vi "SelectSpectrum.vi"(4 "Following":enum32{"Mag", "Temp", "Last"}(radio), 6 "Param":enum16{"S11", "S21", "S12", "S22"}(ring), 8 "Cursor.Cursor Index":i32, 10 "Data_IN":T1={"Value"=0.0, "GUI Data Cluster"={"S11"=FALSE, "S21"=FALSE, "S12"=FALSE, "S22"=FALSE, "S11Meas"=enum."Log-magnitude (dB)", "S21Meas"=enum."Log-magnitude (dB)", "S12Meas"=enum."Log-magnitude (dB)", "S22Meas"=enum."Log-magnitude (dB)", "S11Param"=enum."S11", "S21Param"=enum."S21", "S12Param"=enum."S12", "S22Param"=enum."S22"}, "Timing"={"Last Operation"=0.0, "Stop @ T/B"=FALSE, "Last Temp"=0.0, "Last Mag"=0.0, "Ramp Param"={"End T (K)"=0.0, "Delta T (K)"=0.0, "End B (T)"=0.0, "Delta B (T)"=0.0}, "LastOp?"=FALSE, "FirstOp?"=FALSE}, "Measurements"=[], "Hardware"={"VNA TCP Con"=refnum, "VNA TCP Port"=5025, "Global T VAR"="", "Global B VAR"=""}, "Operation"={"Operation Mode"=enum."Logging", "Log Folder"=path "", "Measure Mode"=enum."Deltat"}}) -> (1 "VNA Out":cluster{"Ramp Pattern":dbl[], "VNA S22":dbl[]}, 2 "Data_Out":T1={"Value"=0.0, "GUI Data Cluster"={"S11"=FALSE, "S21"=FALSE, "S12"=FALSE, "S22"=FALSE, "S11Meas"=enum."Log-magnitude (dB)", "S21Meas"=enum."Log-magnitude (dB)", "S12Meas"=enum."Log-magnitude (dB)", "S22Meas"=enum."Log-magnitude (dB)", "S11Param"=enum."S11", "S21Param"=enum."S21", "S12Param"=enum."S12", "S22Param"=enum."S22"}, "Timing"={"Last Operation"=0.0, "Stop @ T/B"=FALSE, "Last Temp"=0.0, "Last Mag"=0.0, "Ramp Param"={"End T (K)"=0.0, "Delta T (K)"=0.0, "End B (T)"=0.0, "Delta B (T)"=0.0}, "LastOp?"=FALSE, "FirstOp?"=FALSE}, "Measurements"=[], "Hardware"={"VNA TCP Con"=refnum, "VNA TCP Port"=5025, "Global T VAR"="", "Global B VAR"=""}, "Operation"={"Operation Mode"=enum."Logging", "Log Folder"=path "", "Measure Mode"=enum."Deltat"}})   [LabVIEW 2021]
uses:
  Sources/Data_Cluster.ctl
  Sources/Measurement_Cluster.ctl
  Sources/Mode_Enum.ctl
  <vilib>/Analysis/1siggen.llb/Ramp Pattern by Samples.vi
  <vilib>/Analysis/NI_AALBase.lvlib
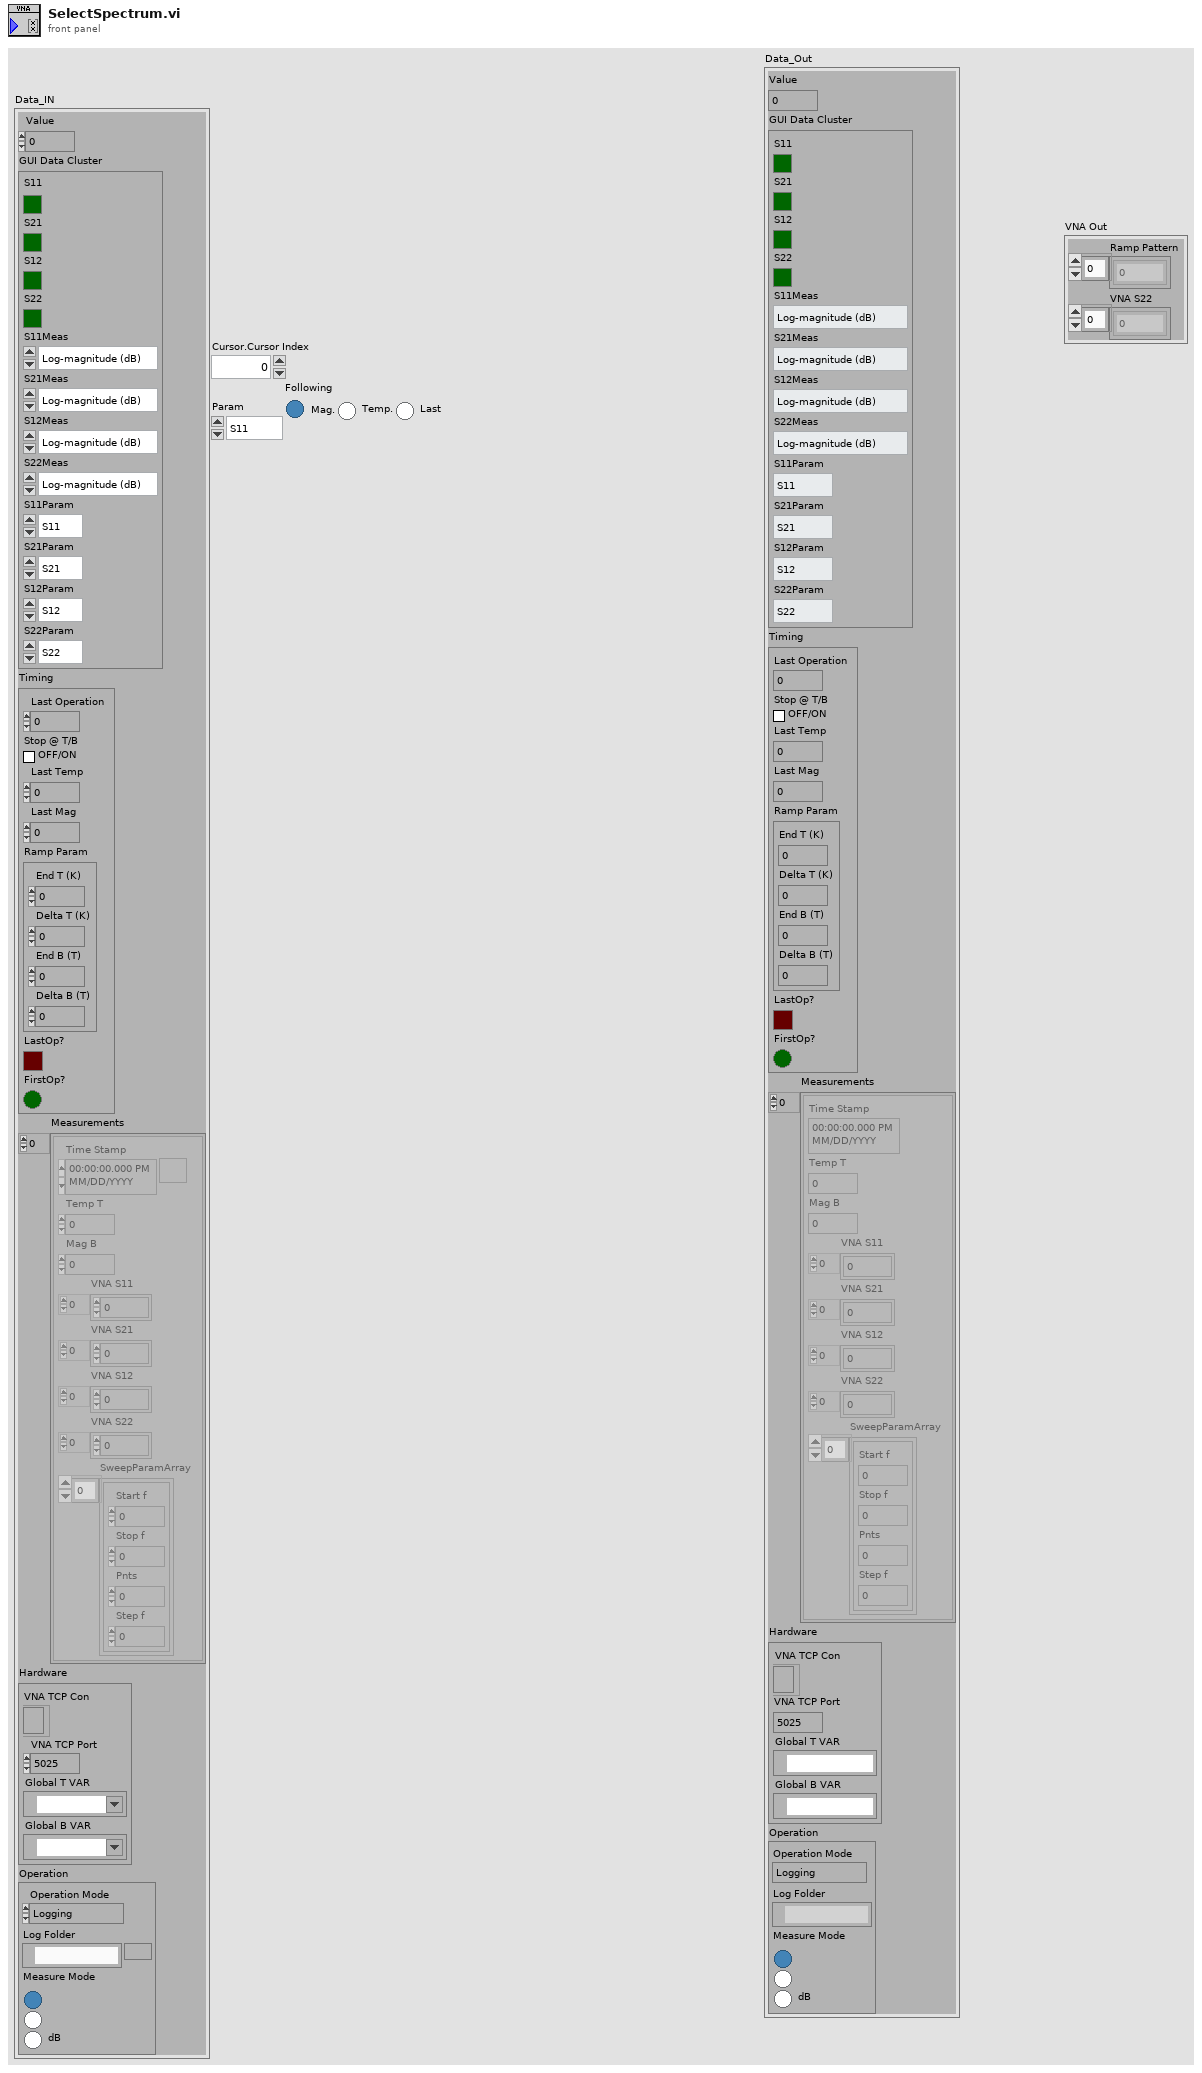
[diagram p1: front panel]
types:
  T1 = typedef "Data_Cluster.ctl" = cluster{"Value":dbl, "GUI Data Cluster":cluster{"S11":bool, "S21":bool, "S12":bool, "S22":bool, "S11Meas":enum16{"Log-magnitude (dB)", "Linear magnitude", "Phase (deg)", "Time Domain", "Real", "Imaginary", "Group Delay", "Polarlinear"}, "S21Meas":enum16{"Log-magnitude (dB)", "Linear magnitude", "Phase (deg)", "Time Domain", "Real", "Imaginary", "Group Delay", "Polarlinear"}, "S12Meas":enum16{"Log-magnitude (dB)", "Linear magnitude", "Phase (deg)", "Time Domain", "Real", "Imaginary", "Group Delay", "Polarlinear"}, "S22Meas":enum16{"Log-magnitude (dB)", "Linear magnitude", "Phase (deg)", "Time Domain", "Real", "Imaginary", "Group Delay", "Polarlinear"}, "S11Param":enum16{"S11", "S21", "S12", "S22"}, "S21Param":enum16{"S11", "S21", "S12", "S22"}, "S12Param":enum16{"S11", "S21", "S12", "S22"}, "S22Param":enum16{"S11", "S21", "S12", "S22"}}, "Timing":cluster{"Last Operation":dbl, "Stop @ T/B":bool, "Last Temp":dbl, "Last Mag":dbl, "Ramp Param":cluster{"End T (K)":dbl, "Delta T (K)":dbl, "End B (T)":dbl, "Delta B (T)":dbl}, "LastOp?":bool, "FirstOp?":bool}, "Measurements":T2[], "Hardware":cluster{"VNA TCP Con":refnum<k5>, "VNA TCP Port":i32, "Global T VAR":refnum<k21>, "Global B VAR":refnum<k21>}, "Operation":cluster{"Operation Mode":T3, "Log Folder":path, "Measure Mode":enum32{"Deltat", "DeltaT", "dB"}}}
  T2 = typedef "Measurement_Cluster.ctl" = cluster{"Time Stamp":timestamp, "Temp T":dbl, "Mag B":dbl, "VNA S11":dbl[], "VNA S21":dbl[], "VNA S12":dbl[], "VNA S22":dbl[], "SweepParamArray":cluster{"Start f":dbl, "Stop f":dbl, "Pnts":i32, "Step f":dbl}[]}
  T3 = typedef "Mode_Enum.ctl" = enum16{"Logging", "Idle-Off", "Idle"}
  T4 = cluster{"Start f":dbl, "Stop f":dbl, "Pnts":i32, "Step f":dbl}[]
  T5 = cluster{"Start f":dbl, "Stop f":dbl, "Pnts":i32, "Step f":dbl}
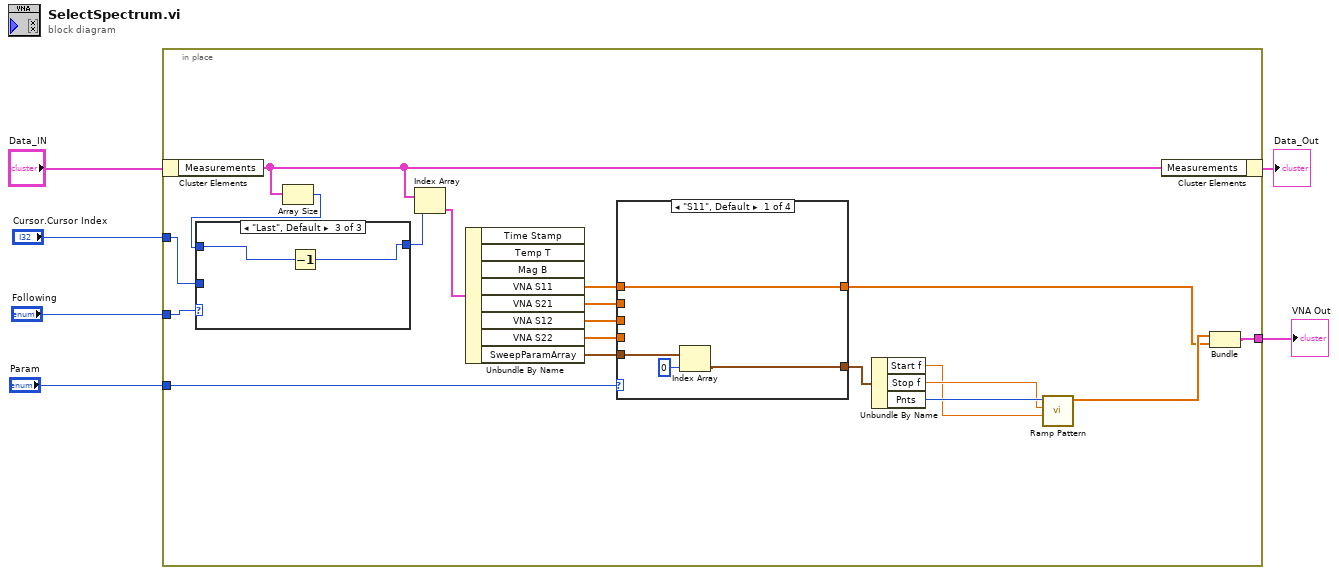
[diagram p0: block diagram]
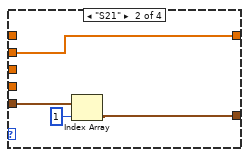
[diagram p4: hidden frame]
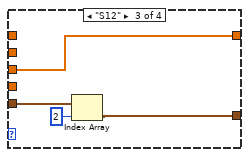
[diagram p5: hidden frame]
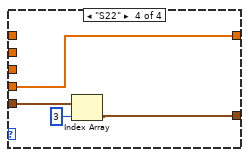
[diagram p6: hidden frame]
diagram:
  n1 = in-place {
    in-place-border: "Cursor.Cursor Index" -> [w10]
    in-place-border: "Param" -> [w25]
    in-place-border: [w12] -> w2
    in-place-border: "Following" -> [w11]
    n2 = in-place-cluster #1("Data_IN") -> ("Measurements"=w9:T2[])
    n3 = Array Size(array=w9) -> (size(s)=w8:i32)
    n4 = case shown="\"Last\", Default" w11 {
      tunnel: w10 -> [w26 w27 _]
      tunnel: w8 -> [_ _ w29]
      tunnel: [w26 w27 w28] -> w7
      frame "Temp" {
      }
      frame "Mag" {
      }
      frame "Last", Default {
        n5 = Decrement(x=w29) -> (x-1=w28:i32)
      }
    }
    n6 = Index Array(array=w9, index=w7) -> (element=w24:T2)
    n7 = Unbundle By Name(w24) -> ("VNA S11"=w23:dbl[], "VNA S21"=w21:dbl[], "VNA S12"=w20:dbl[], "VNA S22"=w19:dbl[], "SweepParamArray"=w22:T4)  [unwired: 3 out]
    n8 = case shown="\"S11\", Default" w25 {
      tunnel: w23 -> [w32 _ _ _]
      tunnel: w22 -> [w33 w37 w41 w45]
      tunnel: [w32 w34 w38 w42] -> w13
      tunnel: [w31 w36 w40 w44] -> w18
      tunnel: w21 -> [_ w34 _ _]
      tunnel: w20 -> [_ _ w38 _]
      tunnel: w19 -> [_ _ _ w42]
      frame "S11", Default {
        n9 = Index Array(array=w33, index=0) -> (element=w31:T5)
      }
      frame "S21" {
        n10 = Index Array(array=w37, index=1) -> (element=w36:T5)
      }
      frame "S12" {
        n11 = Index Array(array=w41, index=2) -> (element=w40:T5)
      }
      frame "S22" {
        n12 = Index Array(array=w45, index=3) -> (element=w44:T5)
      }
    }
    n13 = Unbundle By Name(w18) -> ("Start f"=w15:dbl, "Stop f"=w16:dbl, "Pnts"=w17:i32)
    n14 = call-poly <vilib>:"Ramp Pattern.vi"("start"=w15, "end"=w16, "samples"=w17) -> ("Ramp Pattern"=w14:dbl[])  [unwired: 7 in, 1 out]
    n15 = in-place-cluster #1("Measurements"=w9) -> (→"Data_Out":T1)
    n16 = Bundle("Ramp Pattern"=w14, "VNA S22"=w13) -> (w12:cluster{"Ramp Pattern":dbl[], "VNA S22":dbl[]})  [unwired: 1 in]
  }
  "VNA Out" <- w2
